vi "Do.vi"(8 "error in (no error)":errorcluster, 10 "Actor in":refnum<class "Actor.lvclass">, 11 "GetMessage Msg":refnum<class "GetMessage Msg.lvclass">) -> (0 "error out":errorcluster, 2 "Actor out":refnum<class "Actor.lvclass">)   [LabVIEW 2023, in "TCP_Server_Connection_Handler.lvlib" / "GetMessage Msg.lvclass"]
doc: "This VI delivers the message to the actor by calling the appropriate method(s) on the actor."
uses:
  GetMessage Msg.lvclass
  GetMessage Msg.lvclass/GetMessage Msg.ctl
  f8963acf-0c52-4e96-8a53-7aee5a4d43d9.vi
  TCP_Server_Connection_Handler/TCP_Server_Connection_Handler.lvclass
  <vilib>/ActorFramework/Actor/Actor.lvclass
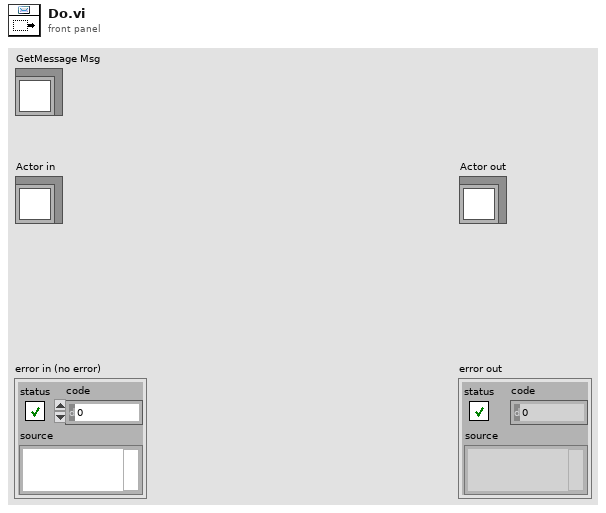
[diagram p1: front panel]
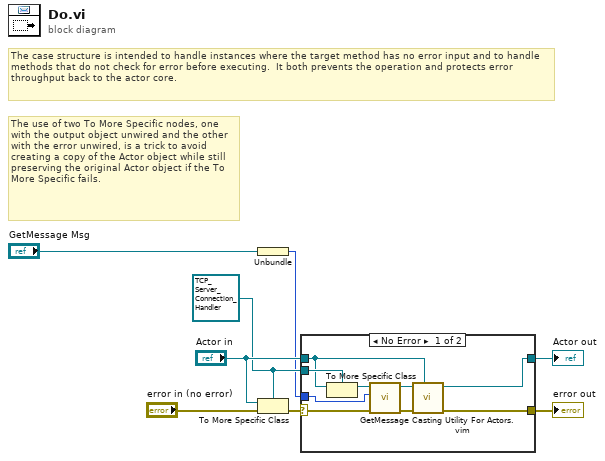
[diagram p0: block diagram]
diagram:
  w3 = refnum<class "TCP_Server_Connection_Handler.lvclass"> refnum ("Actor in")
  # "The use of two To More Specific nodes, one with the output object unwired and the other with the error unwired, is a trick to avoid creating a copy of the Actor object while still preserving the original Actor object if the To More Specific fails."
  # "The case structure is intended to handle instances where the target method has no error input and to handle methods that do not check for error before executing.  It both prevents the operation and protects error throughput back to the actor core."
  n1 = Unbundle("GetMessage Msg") -> (w1:i32)
  n2 = To More Specific Class(target class=w3, reference="Actor in", error in="error in (no error)") -> (error out=w2:errorcluster)  [unwired: 1 out]
  n3 = case shown="No Error" w2 {
    selector: w2 -> [w17 w19]
    tunnel: [w11 w19] -> w8
    tunnel: [w12 w18] -> w7
    tunnel: "Actor in" -> [w14 w18]
    tunnel: w3 -> [w15 _]
    tunnel: w1 -> [w9 _]
    frame No Error {
      n4 = To More Specific Class(target class=w15, reference=w14) -> (specific class reference=w16:refnum<class "TCP_Server_Connection_Handler.lvclass">)  [unwired: 1 in, 1 out]
      n5 = call "GetMessage.vi"("error in (no error)"=w17, "Message length"=w9, "TCP_Server_Connection_Handler in"=w16) -> ("error out"=w10:errorcluster, "TCP_Server_Connection_Handler out"=w13:refnum<class "TCP_Server_Connection_Handler.lvclass">)  [unwired: 7 in]
      n6 = call "Casting Utility For Actors.vim"("type"=w14, "error in (no error)"=w10, "Actor in"=w13) -> ("error out"=w11:errorcluster, "Actor out"=w12:refnum<class "Actor.lvclass">)  [unwired: 7 in]
    }
    frame Error {
      # "If type check fails, pass the original object out again."
    }
  }
  "error out" <- w8
  "Actor out" <- w7
